vi "Referee.vi"(0 "element":u8[](array[numeric])) -> (4 "output cluster":T1, 15 "error out":errorcluster)   [LabVIEW 2023]
uses:
  Controls/SSL Referee.ctl
  SSL Referee Team Info.ctl
  Varint Decoder uint64.vi
  Varint Decoder uint32.vi
panel:
  in  "error in":errorcluster
  out "error out 3":errorcluster
  in  "error in 2":errorcluster
  out "error out 2":errorcluster
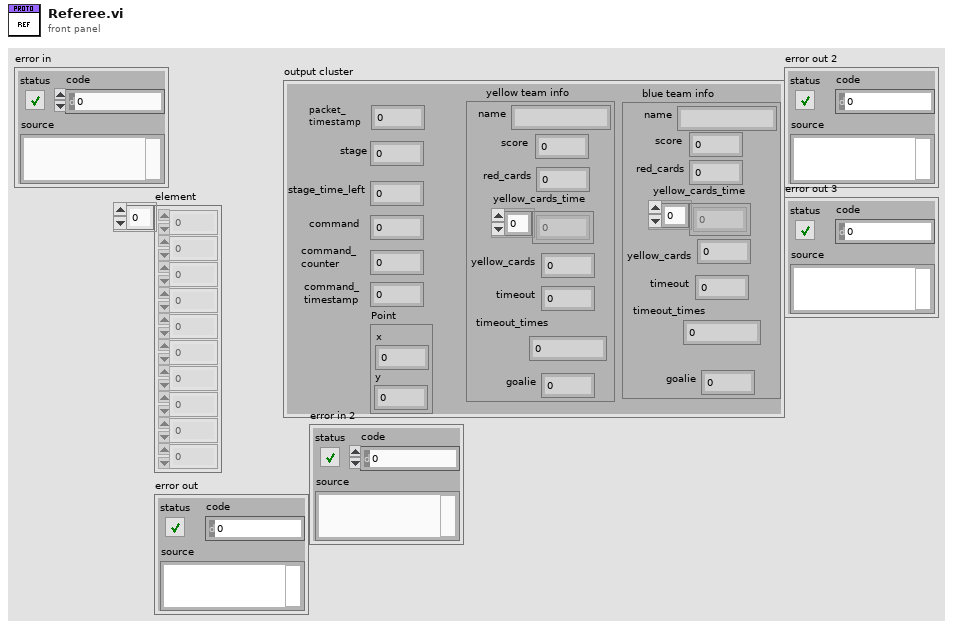
[diagram p1: front panel]
types:
  T1 = typedef "SSL Referee.ctl" = cluster{"packet_\ntimestamp":u64, "stage":u64, "stage_time_left":i32, "command ":u64, "command_\ncounter ":u32, "command_\ntimestamp":u64, "yellow team info":T2, "blue team info":T2, "Point":cluster{"x":sgl, "y":sgl}}
  T2 = typedef "SSL Referee Team Info.ctl" = cluster{"name":string, "score":u32, "red_cards":u32, "yellow_cards_time":u32[], "yellow_cards":u32, "timeout":u32, "timeout_times":u32, "goalie":u32}
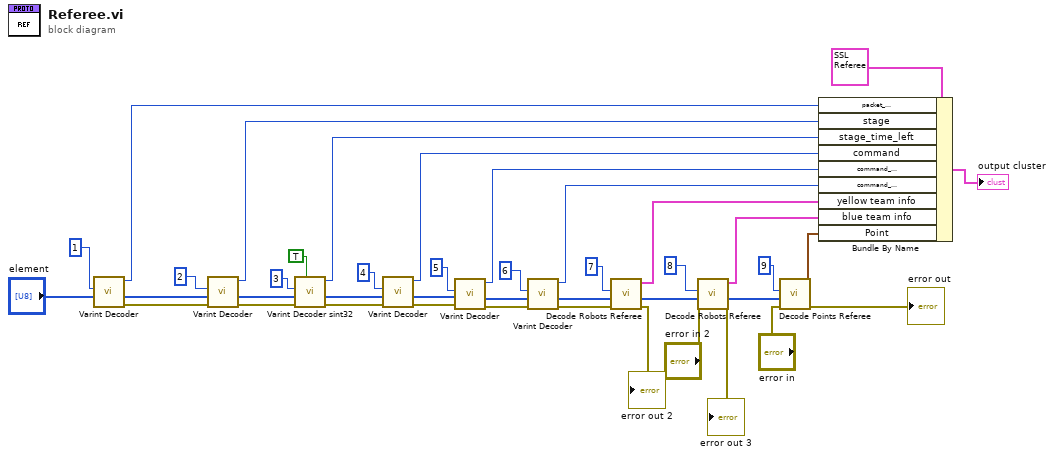
[diagram p0: block diagram]
diagram:
  n1 = call-poly "Varint Decoder.vi"("Array"="element", "Key"=1) -> ("error out"=w22:errorcluster, "array w/ subset deleted"=w20:u8[], "Varint"=w18:u64)  [unwired: 6 in, 1 out]
  n2 = call-poly "Varint Decoder.vi"("error in (no error)"=w22, "Array"=w20, "Key"=2) -> ("error out"=w25:errorcluster, "array w/ subset deleted"=w26:u8[], "Varint"=w17:u64)  [unwired: 5 in, 1 out]
  n3 = call "Varint Decoder sint32.vi"("Optional"=TRUE, "error in (no error)"=w25, "Array"=w26, "Key"=3) -> ("error out"=w28:errorcluster, "array w/ subset deleted"=w29:u8[], "Varint"=w16:i32)  [unwired: 4 in, 1 out]
  n4 = call-poly "Varint Decoder.vi"("error in (no error)"=w28, "Array"=w29, "Key"=4) -> ("error out"=w31:errorcluster, "array w/ subset deleted"=w33:u8[], "Varint"=w15:u64)  [unwired: 5 in, 1 out]
  n5 = call-poly "Varint Decoder.vi"("error in (no error)"=w31, "Array"=w33, "Key"=5) -> ("error out"=w32:errorcluster, "array w/ subset deleted"=w34:u8[], "Varint"=w14:u32)  [unwired: 5 in, 1 out]
  n6 = call-poly "Varint Decoder.vi"("error in (no error)"=w32, "Array"=w34, "Key"=6) -> ("error out"=w37:errorcluster, "array w/ subset deleted"=w38:u8[], "Varint"=w13:u64)  [unwired: 5 in, 1 out]
  n7 = call "Decode Robots Referee.vi"("error in"=w37, "array"=w38, "Key"=7) -> ("error out"=→"error out 2":errorcluster, "array w/ subset deleted out"=w39:u8[], "team info"=w12:T2)  [unwired: 6 in]
  n8 = call "Decode Robots Referee.vi"("error in"="error in 2", "array"=w39, "Key"=8) -> ("error out"=→"error out 3":errorcluster, "array w/ subset deleted out"=w9:u8[], "team info"=w11:T2)  [unwired: 6 in]
  n9 = call "Decode Points Referee.vi"("error in"="error in", "array"=w9, "Key"=9) -> ("error out"=→"error out":errorcluster, "Point"=w5:cluster{"x":sgl, "y":sgl})  [unwired: 6 in, 1 out]
  n10 = Bundle By Name(cluster=T1 {"packet_\ntimestamp"=0, "stage"=0, "stage_time_left"=0, "command "=0, "command_\ncounter "=0, "command_\ntimestamp"=0, "yellow team info"={"name"="", "score"=0, "red_cards"=0, "yellow_cards_time"=[], "yellow_cards"=0, "timeout"=0, "timeout_times"=0, "goalie"=0}, "blue team info"={"name"="", "score"=0, "red_cards"=0, "yellow_cards_time"=[], "yellow_cards"=0, "timeout"=0, "timeout_times"=0, "goalie"=0}, "Point"={"x"=0.0, "y"=0.0}} ("output cluster"), "packet_\ntimestamp"=w18, "stage"=w17, "stage_time_left"=w16, "command"=w15, "command_\ncounter"=w14, "command_\ntimestamp"=w13, "yellow team info"=w12, "blue team info"=w11, "Point"=w5) -> (→"output cluster":T1)
